vi "Load Configuration.vi"(8 "error in":errorcluster) -> (0 "error out":errorcluster, 3 "Theme Config out":refnum<class "Theme Config.lvclass">)   [LabVIEW 2021, in "Theme Config.lvclass"]
uses:
  Theme Config.lvclass
  C:/Program Files (x86)/National Instruments/LabVIEW 2021/vi.lib/JDP Science/JSONtext/Config Files/Config File.lvclass
  <vilib>/JDP Science/JSONtext/Config Files/Config File.lvclass/Config File.ctl
  3b317bd2-2840-4331-bfb7-99d377f3c52f.vi
  <vilib>/JDP Science/JSONtext/JSON text to Variant.vi
  <vilib>/JDP Science/JSONtext/LVClass Serializer/JSONtext LVClass Serializer.lvclass
  Theme Config.lvclass/Theme Config.ctl
  <vilib>/JDP Science/JSONtext/Config Files/Config File.lvclass
  <vilib>/JDP Science/JSONtext/JSONtext.lvlib
  Theme Serializer/Theme Serializer.lvclass
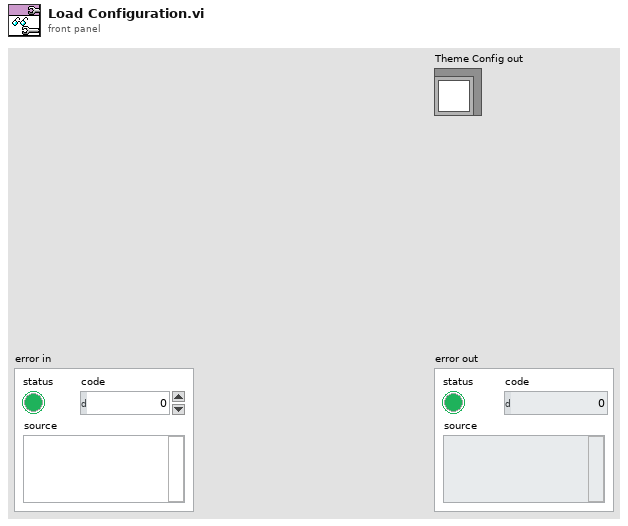
[diagram p1: front panel]
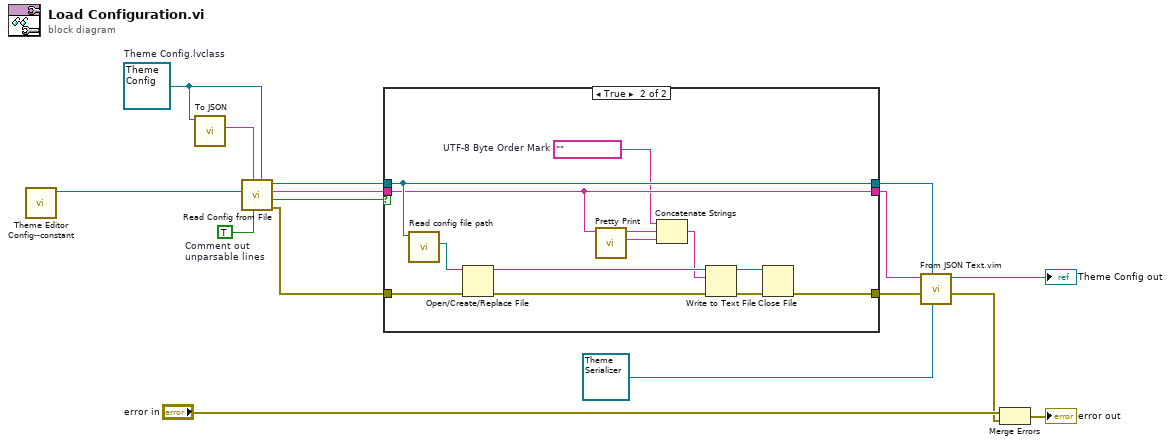
[diagram p0: block diagram]
diagram:
  w11 = TRUE  # Comment out unparsable lines
  w14 = refnum<class "Theme Config.lvclass"> refnum  # Theme Config.lvclass
  n1 = call "Theme Editor Config--constant.vi"() -> ("Button Editor Config"=w12:path)  [unwired: 11 in]
  n2 = call "To JSON.vi"("Theme Config in"=w14) -> ("JSON"=w13:string)  [unwired: 8 in, 2 out]
  n3 = call <vilib>:"Read Config from File.vi"("Config File (type)"=w14, "Comment out unparsable lines"=w11, "Template (JSON Object)"=w13, "config file path"=w12) -> ("error out"=w9:errorcluster, "Template Used (file missing or corrupted)"=w10:bool, "<JSON>Config"=w8:string, "Config File"=w7:refnum<class "Theme Config.lvclass">)  [unwired: 4 in]
  n4 = case shown="True" w10 {
    tunnel: w9 -> [w19 w32]
    tunnel: w8 -> [w18 w27]
    tunnel: w7 -> [w17 w31]
    tunnel: [w17 w31] -> w4
    tunnel: [w18 w27] -> w5
    tunnel: [w19 w20] -> w6
    frame False {
    }
    frame True {
      w24 = "﻿"  # UTF-8 Byte Order Mark
      n5 = call <vilib>:"Read config file path.vi"("Config File in"=w31) -> ("config file path"=w30:path)  [unwired: 10 in]
      n6 = Open/Create/Replace File(file path (use dialog)=w30, error in=w32) -> (refnum out=w28:refnum<file>, error out=w29:errorcluster)  [unwired: 4 in, 1 out]
      n7 = call <vilib>:"Pretty Print.vi"("JSON"=w27) -> ("Rest of Input String"=w26:string, "<JSON>"=w25:string)  [unwired: 8 in, 1 out]
      n8 = Concatenate Strings(w24, w25, w26) -> (w23:string)
      n9 = Write to Text File(file (use dialog)=w28, text=w23, error in=w29) -> (refnum out=w21:refnum<file>, error out=w22:errorcluster)  [unwired: 1 in, 1 out]
      n10 = Close File(refnum=w21, error in=w22) -> (error out=w20:errorcluster)  [unwired: 1 out]
    }
  }
  n11 = call "From JSON Text.vim"("LVClass Serializer"=refnum<class "Theme Serializer.lvclass"> refnum ("Theme Serializer.lvclass"), "Data Type and Default Value"=w4, "error in (no error)"=w6, "JSON"=w5) -> ("error out"=w2:errorcluster, "Data out"=→"Theme Config out":refnum<class "Theme Config.lvclass">)  [unwired: 6 in]
  n12 = Merge Errors("error in", w2) -> (→"error out":errorcluster)
